vi "Close GMAP References.vi"(8 "error in (no error)":errorcluster) -> (0 "error out":errorcluster)   [LabVIEW 2014]
uses:
  Reference/SubVI/Mini Map DLL Refernce.vi
  Reference/SubVI/GMap DLL Refernce.vi
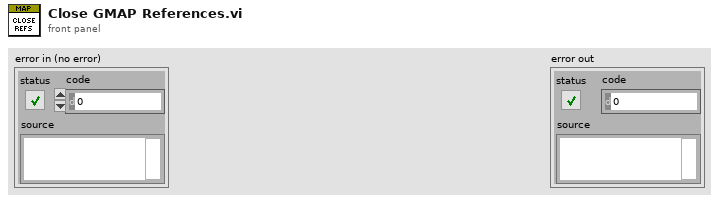
[diagram p1: front panel]
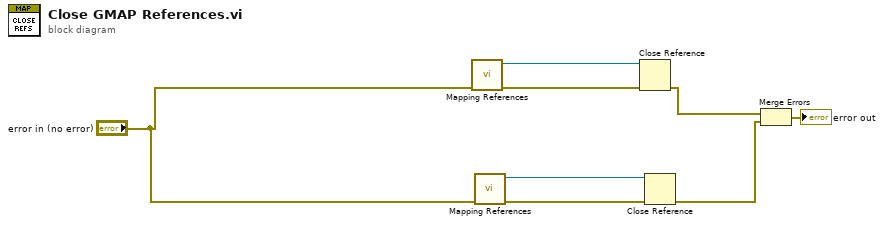
[diagram p0: block diagram]
diagram:
  n1 = call-poly "Mapping References.vi"("Error In"="error in (no error)") -> ("Error Out"=w1:errorcluster, "GMap DLL Reference"=w5:refnum<k24>)  [unwired: 9 in]
  n2 = call-poly "Mapping References.vi"("Error In"="error in (no error)") -> ("Error Out"=w2:errorcluster, "Mini Map DLL Reference"=w4:refnum<k24>)  [unwired: 9 in]
  n3 = Close Reference(reference=w5, error in (no error)=w1) -> (error out=w8:errorcluster)
  n4 = Close Reference(reference=w4, error in (no error)=w2) -> (error out=w7:errorcluster)
  n5 = Merge Errors(w8, w7) -> (→"error out":errorcluster)
